vi "tm484_DSP.vi"() -> ()   [LabVIEW 2023, in "HamamatsuCam.lvlib" / "HamamatsuCam.lvclass"]
uses:
  HamamatsuCam/HamamatsuCam/HamamatsuCam.lvclass
panel:
  in  "SC Enable":bool
  in  "BG Enable":bool
  in  "Frame Averaging":i32(ring)=1 items=["1 Frame"=1, "2 Frames"=2, "4 Frames"=4]
  in  "Recursive Frames":i32(ring)=1 items=["1 Frame"=1, "2 Frames"=2, "4 Frames"=4, "8 Frames"=8, "16 Frames"=16]
  out "Image":u16[][](graph)
  in  "Quit":bool
  out "Error Out":errorcluster {"code" format="%.0x"}
  # "This is an example how to use the DSP functions.\nNot all camera have the DSP functions. Please\ncheck your camera manual to see your camera's\ncapabilities."
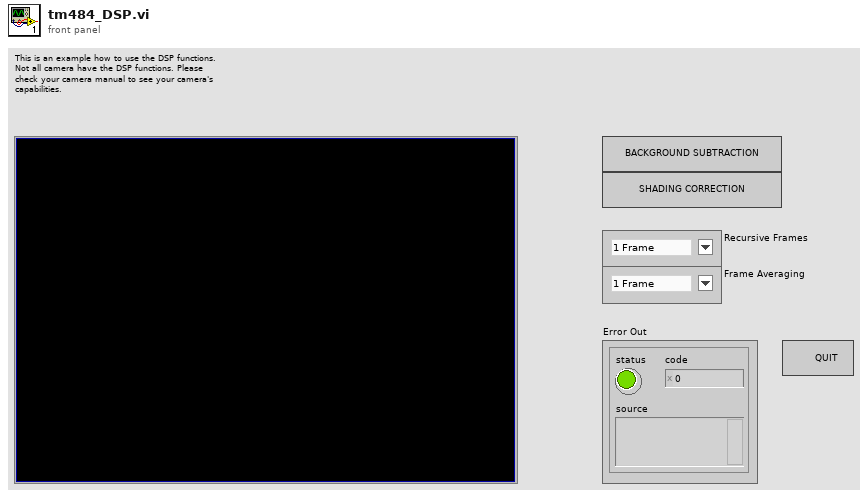
[diagram p1: front panel]
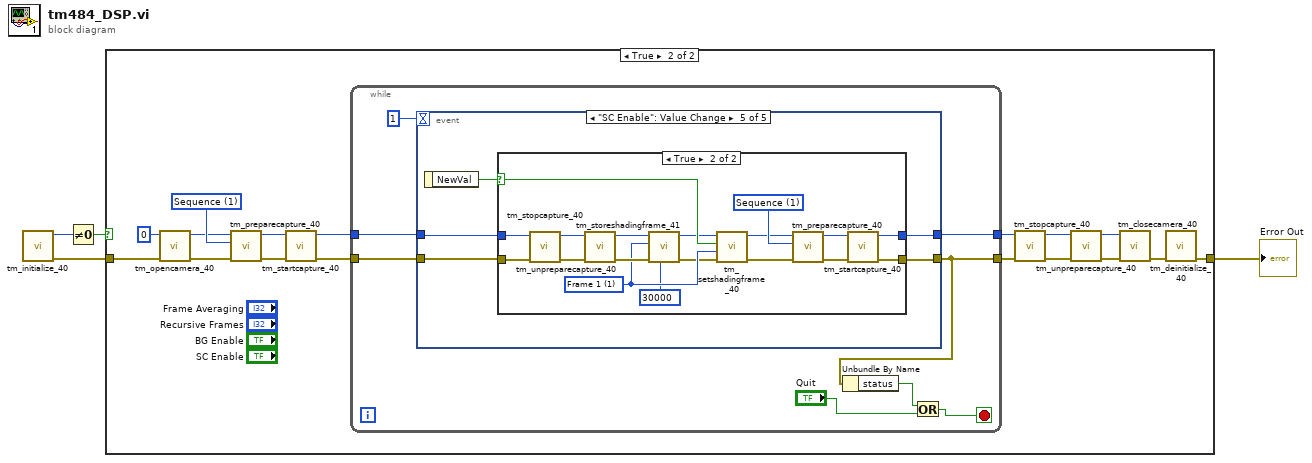
[diagram p0: block diagram]
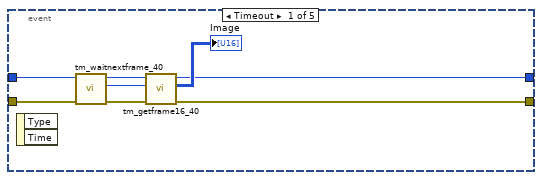
[diagram p3: hidden frame]
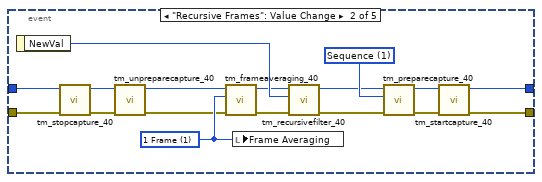
[diagram p4: hidden frame]
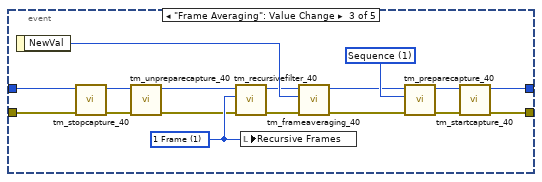
[diagram p5: hidden frame]
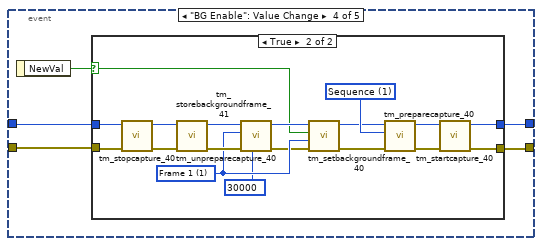
[diagram p6: hidden frame]
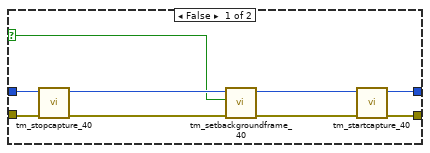
[diagram p7: hidden frame]
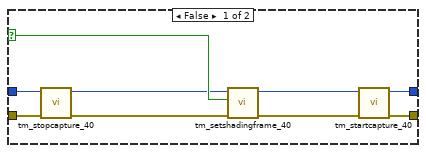
[diagram p8: hidden frame]
diagram:
  n1 = call "tm_initialize_40.vi"() -> ("error out"=w1:errorcluster, "Number Of Cameras"=w2:u32)  [unwired: 8 in, 2 out]
  n2 = Not Equal To 0?(x=w2) -> (x != 0?=w4:bool)
  n3 = case shown="True" w4 {
    tunnel: w1 -> [w5 w22]
    tunnel: [w5 w19] -> w3
    frame False {
    }
    frame True {
      w12 = 1 items=["Snap", "Sequence"] ("Capture mode")
      n4 = call "tm_opencamera_40.vi"("error in (no error)"=w22, "Camera Index"=u32 0) -> ("error out"=w9:errorcluster, "Handle out"=w8:u32)  [unwired: 7 in, 1 out]
      n5 = call "tm_preparecapture_40.vi"("error in (no error)"=w9, "Capture mode"=w12, "Handle in"=w8) -> ("error out"=w10:errorcluster, "Handle out"=w11:u32)  [unwired: 5 in, 2 out]
      n6 = call "tm_startcapture_40.vi"("error in (no error)"=w10, "Handle in"=w11) -> ("error out"=w6:errorcluster, "Handle out"=w7:u32)  [unwired: 8 in]
      n7 = while {
        tunnel: [w28] -> w15
        tunnel: [w24] -> w16
        tunnel: w7 -> [w30]
        tunnel: w6 -> [w29]
        stop <- w23 stop-if-true
        n8 = event shown="[4] \"SC Enable\": Value Change" {
          selector: _ -> [_ _ _ _ _]
          dyn-events: _ -> [_ _ _ _ _]
          timeout: 1 -> [_ _ _ _ _]
          tunnel: w30 -> [w34 w47 w64 w77 w108]
          tunnel: w29 -> [w33 w48 w63 w76 w107]
          tunnel: [w31 w39 w57 w75 w106] -> w28
          tunnel: [w32 w40 w56 w74 w105] -> w24
          event Timeout {
            n9 = event-data() -> ()  [unwired: 1 in, 2 out]
            n10 = call "tm_waitnextframe_40.vi"("error in (no error)"=w33, "Handle in"=w34) -> ("error out"=w36:errorcluster, "Frame Index"=w38:i32, "Handle out"=w35:u32)  [unwired: 6 in, 1 out]
            n11 = call "tm_getframe16_40.vi"("error in (no error)"=w36, "Frame Index"=w38, "Handle in"=w35) -> ("error out"=w32:errorcluster, "Data"=→"Image":u16[][], "Handle out"=w31:u32)  [unwired: 5 in, 1 out]
          }
          event "Recursive Frames": Value Change {
            w43 = 1 items=["Snap", "Sequence"] ("Capture mode")
            w52 = 1 items=["1 Frame"=1, "2 Frames"=2, "4 Frames"=4, "8 Frames"=8, "16 Frames"=16] ("Frames")
            n12 = event-data() -> ("NewVal"=w55:i32)  [unwired: 1 in]
            n13 = call "tm_stopcapture_40.vi"("error in (no error)"=w48, "Handle in"=w47) -> ("error out"=w46:errorcluster, "Handle out"=w51:u32)  [unwired: 8 in]
            n14 = call "tm_unpreparecapture_40.vi"("error in (no error)"=w46, "Handle in"=w51) -> ("error out"=w49:errorcluster, "Handle out"=w50:u32)  [unwired: 8 in]
            n15 = call "tm_frameaveraging_40.vi"("error in (no error)"=w49, "Frames"=w52, "Handle in"=w50) -> ("error out"=w53:errorcluster, "Handle out"=w54:u32)  [unwired: 7 in]
            n16 = local write "Frame Averaging"(w52) -> ()
            n17 = call "tm_recursivefilter_40.vi"("error in (no error)"=w53, "Frames"=w55, "Handle in"=w54) -> ("error out"=w42:errorcluster, "Handle out"=w41:u32)  [unwired: 7 in]
            n18 = call "tm_preparecapture_40.vi"("error in (no error)"=w42, "Capture mode"=w43, "Handle in"=w41) -> ("error out"=w45:errorcluster, "Handle out"=w44:u32)  [unwired: 5 in, 2 out]
            n19 = call "tm_startcapture_40.vi"("error in (no error)"=w45, "Handle in"=w44) -> ("error out"=w40:errorcluster, "Handle out"=w39:u32)  [unwired: 8 in]
          }
          event "Frame Averaging": Value Change {
            w60 = 1 items=["Snap", "Sequence"] ("Capture mode")
            w69 = 1 items=["1 Frame"=1, "2 Frames"=2, "4 Frames"=4, "8 Frames"=8, "16 Frames"=16] ("Frames")
            n20 = event-data() -> ("NewVal"=w72:i32)  [unwired: 1 in]
            n21 = call "tm_stopcapture_40.vi"("error in (no error)"=w63, "Handle in"=w64) -> ("error out"=w67:errorcluster, "Handle out"=w68:u32)  [unwired: 8 in]
            n22 = call "tm_unpreparecapture_40.vi"("error in (no error)"=w67, "Handle in"=w68) -> ("error out"=w66:errorcluster, "Handle out"=w65:u32)  [unwired: 8 in]
            n23 = call "tm_recursivefilter_40.vi"("error in (no error)"=w66, "Frames"=w69, "Handle in"=w65) -> ("error out"=w70:errorcluster, "Handle out"=w71:u32)  [unwired: 7 in]
            n24 = local write "Recursive Frames"(w69) -> ()
            n25 = call "tm_frameaveraging_40.vi"("error in (no error)"=w70, "Frames"=w72, "Handle in"=w71) -> ("error out"=w59:errorcluster, "Handle out"=w58:u32)  [unwired: 7 in]
            n26 = call "tm_preparecapture_40.vi"("error in (no error)"=w59, "Capture mode"=w60, "Handle in"=w58) -> ("error out"=w62:errorcluster, "Handle out"=w61:u32)  [unwired: 5 in, 2 out]
            n27 = call "tm_startcapture_40.vi"("error in (no error)"=w62, "Handle in"=w61) -> ("error out"=w56:errorcluster, "Handle out"=w57:u32)  [unwired: 8 in]
          }
          event "BG Enable": Value Change {
            n28 = event-data() -> ("NewVal"=w73:bool)  [unwired: 1 in]
            n29 = case shown="True" w73 {
              selector: w73 -> [w78 w87]
              tunnel: w77 -> [w86 w104]
              tunnel: w76 -> [w85 w103]
              tunnel: [w84 w102] -> w75
              tunnel: [w83 w101] -> w74
              frame False {
                n30 = call "tm_stopcapture_40.vi"("error in (no error)"=w85, "Handle in"=w86) -> ("error out"=w81:errorcluster, "Handle out"=w82:u32)  [unwired: 8 in]
                n31 = call "tm_setbackgroundframe_40.vi"("error in (no error)"=w81, "Enable"=w78, "Handle in"=w82) -> ("error out"=w80:errorcluster, "Handle out"=w79:u32)  [unwired: 7 in]
                n32 = call "tm_startcapture_40.vi"("error in (no error)"=w80, "Handle in"=w79) -> ("error out"=w83:errorcluster, "Handle out"=w84:u32)  [unwired: 8 in]
              }
              frame True {
                w96 = 1 items=["Snap", "Sequence"] ("Capture mode")
                w92 = 1 items=["Frame 1"=1, "Frame 2"=2, "Frame 3"=3, "Frame 4"=4] ("Frame")
                n33 = call "tm_stopcapture_40.vi"("error in (no error)"=w103, "Handle in"=w104) -> ("error out"=w100:errorcluster, "Handle out"=w99:u32)  [unwired: 8 in]
                n34 = call "tm_unpreparecapture_40.vi"("error in (no error)"=w100, "Handle in"=w99) -> ("error out"=w93:errorcluster, "Handle out"=w91:u32)  [unwired: 8 in]
                n35 = call "tm_storebackgroundframe_41.vi"("Timeout"=30000, "error in (no error)"=w93, "Frame"=w92, "Handle in"=w91) -> ("error out"=w90:errorcluster, "Handle out"=w89:u32)  [unwired: 6 in]
                n36 = call "tm_setbackgroundframe_40.vi"("error in (no error)"=w90, "Frame"=w92, "Enable"=w87, "Handle in"=w89) -> ("error out"=w95:errorcluster, "Handle out"=w94:u32)  [unwired: 6 in]
                n37 = call "tm_preparecapture_40.vi"("error in (no error)"=w95, "Capture mode"=w96, "Handle in"=w94) -> ("error out"=w98:errorcluster, "Handle out"=w97:u32)  [unwired: 5 in, 2 out]
                n38 = call "tm_startcapture_40.vi"("error in (no error)"=w98, "Handle in"=w97) -> ("error out"=w101:errorcluster, "Handle out"=w102:u32)  [unwired: 8 in]
              }
            }
          }
          event "SC Enable": Value Change {
            n39 = event-data() -> ("NewVal"=w109:bool)  [unwired: 1 in]
            n40 = case shown="True" w109 {
              selector: w109 -> [w114 w127]
              tunnel: w108 -> [w117 w133]
              tunnel: w107 -> [w118 w134]
              tunnel: [w116 w129] -> w106
              tunnel: [w115 w128] -> w105
              frame False {
                n41 = call "tm_stopcapture_40.vi"("error in (no error)"=w118, "Handle in"=w117) -> ("error out"=w113:errorcluster, "Handle out"=w112:u32)  [unwired: 8 in]
                n42 = call "tm_setshadingframe_40.vi"("error in (no error)"=w113, "Enable"=w114, "Handle in"=w112) -> ("error out"=w110:errorcluster, "Handle out"=w111:u32)  [unwired: 7 in]
                n43 = call "tm_startcapture_40.vi"("error in (no error)"=w110, "Handle in"=w111) -> ("error out"=w115:errorcluster, "Handle out"=w116:u32)  [unwired: 8 in]
              }
              frame True {
                w130 = 1 items=["Snap", "Sequence"] ("Capture mode")
                w122 = 1 items=["Frame 1"=1, "Frame 2"=2, "Frame 3"=3, "Frame 4"=4] ("Frame")
                n44 = call "tm_stopcapture_40.vi"("error in (no error)"=w134, "Handle in"=w133) -> ("error out"=w136:errorcluster, "Handle out"=w135:u32)  [unwired: 8 in]
                n45 = call "tm_unpreparecapture_40.vi"("error in (no error)"=w136, "Handle in"=w135) -> ("error out"=w123:errorcluster, "Handle out"=w124:u32)  [unwired: 8 in]
                n46 = call "tm_storeshadingframe_41.vi"("Timeout"=30000, "error in (no error)"=w123, "Frame"=w122, "Handle in"=w124) -> ("error out"=w121:errorcluster, "Handle out"=w120:u32)  [unwired: 6 in]
                n47 = call "tm_setshadingframe_40.vi"("error in (no error)"=w121, "Frame"=w122, "Enable"=w127, "Handle in"=w120) -> ("error out"=w125:errorcluster, "Handle out"=w126:u32)  [unwired: 6 in]
                n48 = call "tm_preparecapture_40.vi"("error in (no error)"=w125, "Capture mode"=w130, "Handle in"=w126) -> ("error out"=w132:errorcluster, "Handle out"=w131:u32)  [unwired: 5 in, 2 out]
                n49 = call "tm_startcapture_40.vi"("error in (no error)"=w132, "Handle in"=w131) -> ("error out"=w128:errorcluster, "Handle out"=w129:u32)  [unwired: 8 in]
              }
            }
          }
        }
        n50 = Unbundle By Name(w24) -> ("status"=w27:bool)
        n51 = Or(x=w27, y="Quit") -> (x .or. y?=w23:bool)
      }
      n52 = call "tm_stopcapture_40.vi"("error in (no error)"=w16, "Handle in"=w15) -> ("error out"=w13:errorcluster, "Handle out"=w14:u32)  [unwired: 8 in]
      n53 = call "tm_unpreparecapture_40.vi"("error in (no error)"=w13, "Handle in"=w14) -> ("error out"=w18:errorcluster, "Handle out"=w17:u32)  [unwired: 8 in]
      n54 = call "tm_closecamera_40.vi"("error in (no error)"=w18, "Handle in"=w17) -> ("error out"=w20:errorcluster)  [unwired: 9 in]
      n55 = call "tm_deinitialize_40.vi"("error in (no error)"=w20) -> ("error out"=w19:errorcluster)  [unwired: 10 in]
    }
  }
  "Error Out" <- w3
